vi "Lambda Genesys Main Page.vi"(8 "error in (no error)":errorcluster, 11 "Node Ptr":T1 format="%.0x") -> (0 "error out":errorcluster)   [LabVIEW 2011, in "Lambda Genesys2 Custom Device.lvlib"]
uses:
  Lambda Genesys2 Custom Device.lvlib
  <vilib>/NI Veristand/Custom Device API/Custom Device Item Ref.ctl
  Lambda Genesys Device Properties.vi
  <vilib>/NI Veristand/Custom Device API/Get Item Property (String).vi
  <vilib>/NI Veristand/Custom Device API/Get Item Property (I32).vi
  <vilib>/NI Veristand/Custom Device API/Set Item Property (String).vi
  <vilib>/NI Veristand/Custom Device API/Set Item Property (I32).vi
  <vilib>/NI Veristand/Custom Device API/Custom Device API.lvlib
panel:
  in  "Header 2":cluster{"Section Name":string}={"Section Name"="Lambda Genesys Series DC Power Supply"}
  in  "Header":cluster{"Section Name":string}={"Section Name"="Device Settings"}
  in  "Baud Rate":i32(ring)=3 items=["1200", "2400", "4800", "9600", "19200"]
  in  "Address":i32=6
  in  "VISA Resource":string
  in  "Description":string
  in  "Name":string
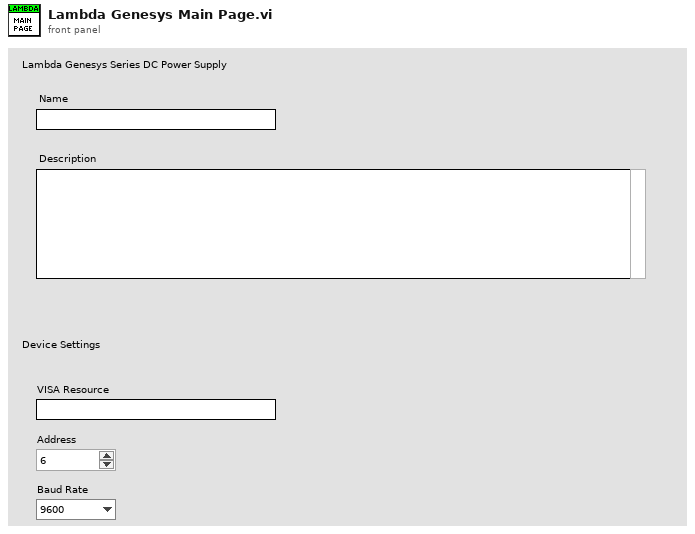
[diagram p1: front panel]
types:
  T1 = typedef "Custom Device API.lvlib/Custom Device Item Ref.ctl" = u64
  T2 = typedef "Custom Device API.lvlib/Custom Device Item Info.ctl" = cluster{"Name":string, "Is Channel":bool, "GUID":string}
  T3 = typedef "Custom Device API.lvlib/Custom Device Commands.ctl" = enum16{"Default", "Item renamed", "Shutdown", "Dynamic button pressed"}
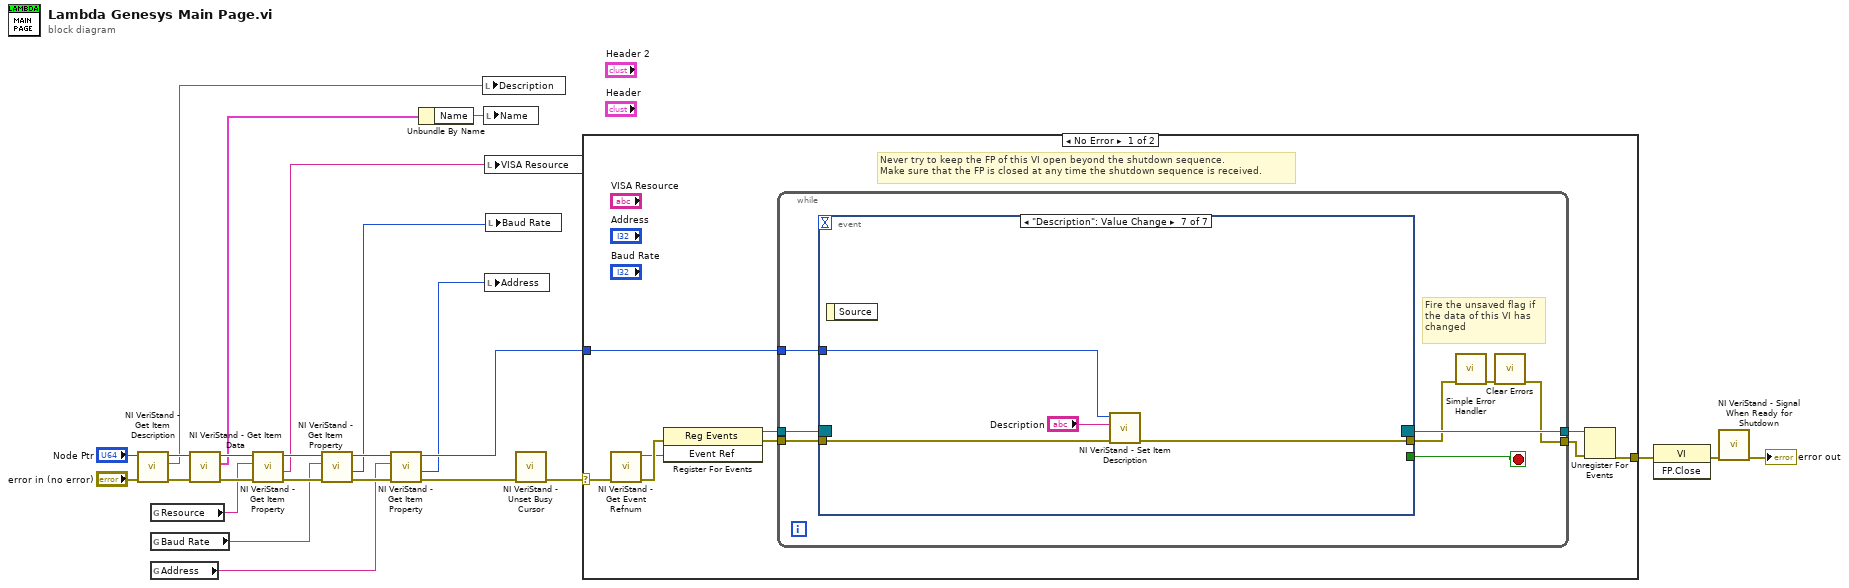
[diagram p0: block diagram]
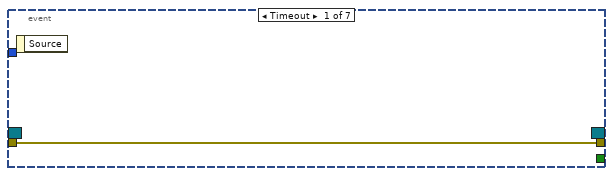
[diagram p2: hidden frame]
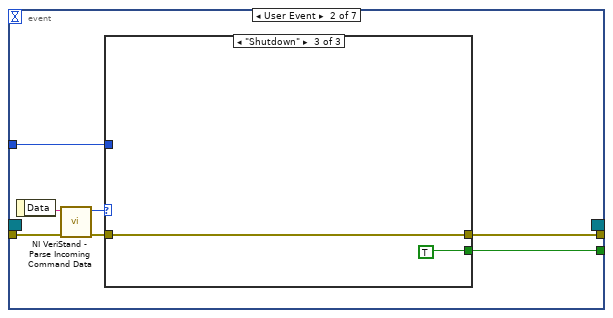
[diagram p3: hidden frame]
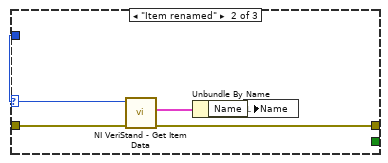
[diagram p5: hidden frame]
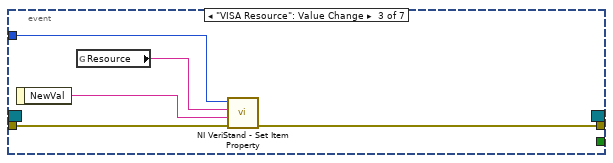
[diagram p6: hidden frame]
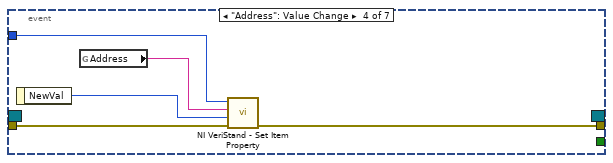
[diagram p7: hidden frame]
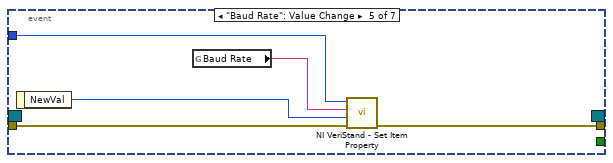
[diagram p8: hidden frame]
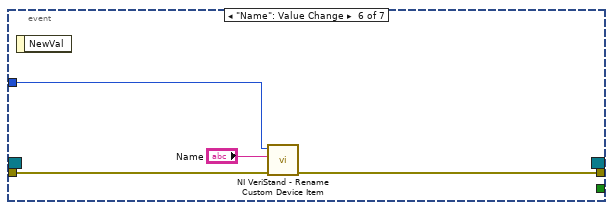
[diagram p9: hidden frame]
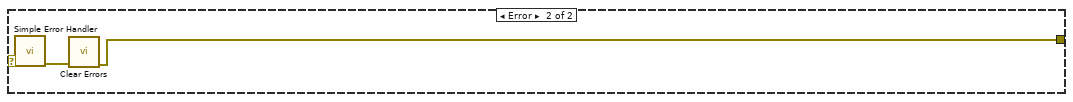
[diagram p10: hidden frame]
diagram:
  n1 = call <vilib>:"NI VeriStand - Get Item Description.vi"("error in (no error)"="error in (no error)", "Item Ref in"="Node Ptr") -> ("error out"=w14:errorcluster, "Description"=w6:string, "Item Ref out"=w13:T1)  [unwired: 7 out]
  n2 = global read "Lambda Genesys Device Properties.vi" "Resource"() -> (w9:string)
  n3 = global read "Lambda Genesys Device Properties.vi" "Baud Rate"() -> (w8:string)
  n4 = global read "Lambda Genesys Device Properties.vi" "Address"() -> (w7:string)
  n5 = call <vilib>:"NI VeriStand - Get Item Data.vi"("error in (no error)"=w14, "Item Ref in"=w13) -> ("error out"=w11:errorcluster, "Item Info"=w5:T2, "Item Ref out"=w10:T1)  [unwired: 7 out]
  n6 = call-poly <vilib>:"NI VeriStand - Get Item Property.vi"("error in (no error)"=w11, "Property Name"=w9, "Item Ref in"=w10) -> ("error out"=w15:errorcluster, "Value"=w3:string, "Item Ref out"=w18:T1)  [unwired: 1 in, 5 out]
  n7 = call-poly <vilib>:"NI VeriStand - Get Item Property.vi"("error in (no error)"=w15, "Property Name"=w8, "Item Ref in"=w18) -> ("error out"=w16:errorcluster, "Value"=w2:i32, "Item Ref out"=w17:T1)  [unwired: 1 in, 5 out]
  n8 = call-poly <vilib>:"NI VeriStand - Get Item Property.vi"("error in (no error)"=w16, "Property Name"=w7, "Item Ref in"=w17) -> ("error out"=w21:errorcluster, "Value"=w1:i32, "Item Ref out"=w19:T1)  [unwired: 1 in, 5 out]
  n9 = Unbundle By Name(w5) -> ("Name"=w12:string)
  n10 = local write "Description"(w6) -> ()
  n11 = local write "Name"(w12) -> ()
  n12 = local write "VISA Resource"(w3) -> ()
  n13 = local write "Address"(w1) -> ()
  n14 = local write "Baud Rate"(w2) -> ()
  n15 = call <vilib>:"NI VeriStand - Unset Busy Cursor.vi"("error in (no error)"=w21) -> ("error out"=w20:errorcluster)  [unwired: 10 out]
  n16 = case shown="No Error" w20 {
    selector: w20 -> [w28 w84]
    tunnel: [w32 w82] -> w25
    tunnel: w19 -> [w29 _]
    frame No Error {
      # "Never try to keep the FP of this VI open beyond the shutdown sequence.\nMake sure that the FP is closed at any time the shutdown sequence is received."
      n17 = call <vilib>:"NI VeriStand - Get Event Refnum.vi"("error in (no error)"=w28) -> ("error out"=w27:errorcluster, "Event Ref"=w26:refnum<user-event>)  [unwired: 9 out]
      n18 = register-events(error in=w27, w26) -> (reference out=w30:refnum<event-registration>, error out=w31:errorcluster)  [unwired: 1 in]
      n19 = while {
        tunnel: [w42] -> w34
        tunnel: [w35] -> w33
        tunnel: w31 -> [w41]
        tunnel: w30 -> [w40]
        tunnel: w29 -> [w38]
        stop <- w39 stop-if-true
        # "Fire the unsaved flag if\nthe data of this VI has\nchanged"
        n20 = event shown="[6] \"Description\": Value Change" {
          selector: w40 -> [_ _ _ _ _ _ _]
          dyn-events: [_ _ _ _ _ _ _] -> w42
          timeout: _ -> [_ _ _ _ _ _ _]
          tunnel: w41 -> [w43 w50 w63 w68 w73 w77 w80]
          tunnel: [_ w46 _ _ _ _ _] -> w39
          tunnel: [w43 w45 w60 w65 w70 w76 w79] -> w37
          tunnel: w38 -> [_ w44 w62 w67 w72 w75 w81]
          event Timeout {
            n21 = event-data() -> ()  [unwired: 2 out]
          }
          event User Event {
            n22 = event-data() -> ("Data"=w49:string)  [unwired: 1 out]
            n23 = call <vilib>:"NI VeriStand - Parse Incoming Command Data.vi"("error in (no error)"=w50, "Incoming data"=w49) -> ("error out"=w48:errorcluster, "Action"=w47:T3)  [unwired: 8 out]
            n24 = case shown="\"Shutdown\"" w47 {
              tunnel: w48 -> [w51 w56 w57]
              tunnel: [_ _ TRUE] -> w46
              tunnel: [w51 w53 w57] -> w45
              tunnel: w44 -> [_ w55 _]
              frame "Default", Default {
              }
              frame "Item renamed" {
                n25 = call <vilib>:"NI VeriStand - Get Item Data.vi"("error in (no error)"=w56, "Item Ref in"=w55) -> ("error out"=w53:errorcluster, "Item Info"=w54:T2)  [unwired: 8 out]
                n26 = Unbundle By Name(w54) -> ("Name"=w52:string)
                n27 = local write "Name"(w52) -> ()
              }
              frame "Shutdown" {
              }
            }
          }
          event "VISA Resource": Value Change {
            n28 = event-data() -> ("NewVal"=w59:string)  [unwired: 1 out]
            n29 = global read "Lambda Genesys Device Properties.vi" "Resource"() -> (w61:string)
            n30 = call-poly <vilib>:"NI VeriStand - Set Item Property.vi"("error in (no error)"=w63, "Value"=w59, "Property Name"=w61, "Item Ref in"=w62) -> ("error out"=w60:errorcluster)  [unwired: 7 out]
          }
          event "Address": Value Change {
            n31 = event-data() -> ("NewVal"=w64:i32)  [unwired: 1 out]
            n32 = global read "Lambda Genesys Device Properties.vi" "Address"() -> (w66:string)
            n33 = call-poly <vilib>:"NI VeriStand - Set Item Property.vi"("error in (no error)"=w68, "Value"=w64, "Property Name"=w66, "Item Ref in"=w67) -> ("error out"=w65:errorcluster)  [unwired: 7 out]
          }
          event "Baud Rate": Value Change {
            n34 = event-data() -> ("NewVal"=w69:i32)  [unwired: 1 out]
            n35 = global read "Lambda Genesys Device Properties.vi" "Baud Rate"() -> (w71:string)
            n36 = call-poly <vilib>:"NI VeriStand - Set Item Property.vi"("error in (no error)"=w73, "Value"=w69, "Property Name"=w71, "Item Ref in"=w72) -> ("error out"=w70:errorcluster)  [unwired: 7 out]
          }
          event "Name": Value Change {
            n37 = event-data() -> ()  [unwired: 2 out]
            n38 = call <vilib>:"NI VeriStand - Rename Custom Device Item.vi"("error in (no error)"=w77, "New Name"="Name", "Item Ref in"=w75) -> ("error out"=w76:errorcluster)  [unwired: 8 out]
          }
          event "Description": Value Change {
            n39 = event-data() -> ()  [unwired: 2 out]
            n40 = call <vilib>:"NI VeriStand - Set Item Description.vi"("error in (no error)"=w80, "Description"="Description", "Item Ref in"=w81) -> ("error out"=w79:errorcluster)  [unwired: 8 out]
          }
        }
        n41 = call <vilib>:"Simple Error Handler.vi"("error in (no error)"=w37) -> ("error out"=w36:errorcluster)  [unwired: 1 in, 7 out]
        n42 = call <vilib>:"Clear Errors.vi"("error in (no error)"=w36) -> ("error out"=w35:errorcluster)  [unwired: 6 out]
      }
      n43 = Unregister For Events(event registration refnum=w34, error in=w33) -> (error out=w32:errorcluster)
    }
    frame Error {
      n44 = call <vilib>:"Simple Error Handler.vi"("error in (no error)"=w84) -> ("error out"=w83:errorcluster)  [unwired: 1 in, 7 out]
      n45 = call <vilib>:"Clear Errors.vi"("error in (no error)"=w83) -> ("error out"=w82:errorcluster)  [unwired: 6 out]
    }
  }
  n46 = invoke class="VI" method="FP.Close"(error in=w25) -> (error out=w24:errorcluster)  [unwired: 2 in, 2 out]
  n47 = call <vilib>:"NI VeriStand - Signal When Ready for Shutdown.vi"("error in (no error)"=w24) -> ("error out"=→"error out":errorcluster)  [unwired: 10 out]
